vi "HowManyLoops.vi"() -> ()   [LabVIEW 2013]
panel:
  in  "Array 4":dbl[](array[numeric])
  in  "Array 3":dbl[](array[numeric])
  in  "Array 2":dbl[](array[numeric])
  in  "Array 1":dbl[](array[numeric])
  out "N":i32
  # "For multiple auto-indexing tunnels, the number of iterations of a for loop is the minimum array length!"
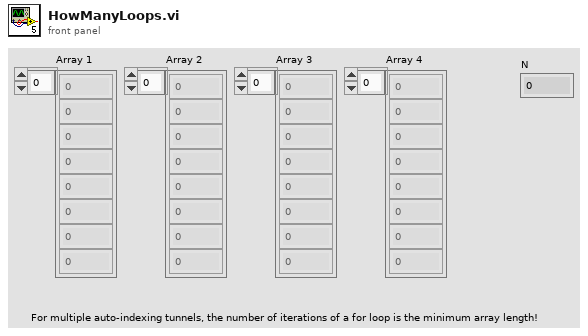
[diagram p1: front panel]
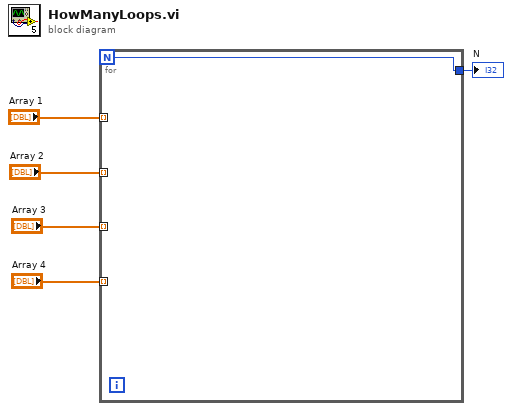
[diagram p0: block diagram]
diagram:
  n1 = for {
    N -> [w6]
    tunnel: [w6] -> w5
    tunnel: "Array 1" -> [_] mode=indexing
    tunnel: "Array 2" -> [_] mode=indexing
    tunnel: "Array 3" -> [_] mode=indexing
    tunnel: "Array 4" -> [_] mode=indexing
  }
  "N" <- w5
